vi "3DS Xray Beam.vi"(10 "FDD":sgl, 11 "DETECTOR SIZE":sgl) -> (3 "XRAY BEAM":T1 {"NormalList"."z" format="%.2f"; "NormalList"."y" format="%.2f"; "NormalList"."x" format="%.2f"; "VertexList"."z" format="%.2f"; "VertexList"."y" format="%.2f"; "VertexList"."x" format="%.2f"})   [LabVIEW 2026, in "XRay Beam.lvclass"]
uses:
  XRay Beam.lvclass
  <vilib>/picture/3D Picture Control/Old 3D Toolkit.llb/model.ctl
  <vilib>/picture/3D Picture Control/Old 3D Toolkit.llb/point3f.ctl
  <vilib>/picture/3D Picture Control/Old 3D Toolkit.llb/VertexMode.ctl
  <vilib>/picture/3D Picture Control/NI_Old 3D Toolkit.lvlib
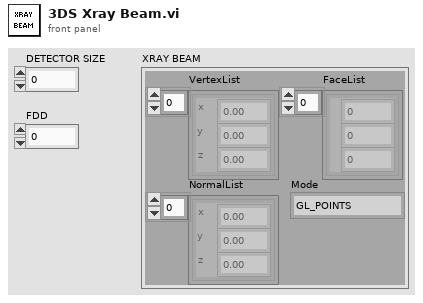
[diagram p1: front panel]
types:
  T1 = typedef "NI_3D Picture Control.lvlib/NI_Old 3D Toolkit.lvlib/model.ctl" = cluster{"VertexList":T2[], "FaceList":cluster{"v1":i32, "v2":i32, "v3":i32}[], "NormalList":T2[], "Mode":T3}
  T2 = typedef "NI_3D Picture Control.lvlib/NI_Old 3D Toolkit.lvlib/point3f.ctl" = cluster{"x":sgl, "y":sgl, "z":sgl}
  T3 = typedef "NI_3D Picture Control.lvlib/NI_Old 3D Toolkit.lvlib/VertexMode.ctl" = enum16{"GL_POINTS", "GL_LINES", "GL_LINE_LOOP", "GL_LINE_STRIP", "GL_TRIANGLES", "GL_TRIANGLE_STRIP", "GL_TRIANGLE_FAN", "GL_QUADS", "GL_QUAD_STRIP", "GL_POLYGON"}
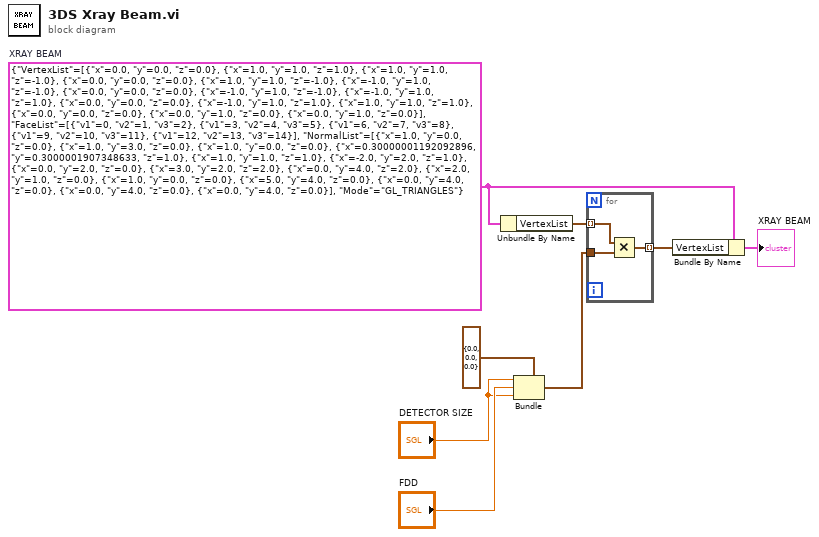
[diagram p0: block diagram]
diagram:
  w1 = T1 {"VertexList"=[{"x"=0.0, "y"=0.0, "z"=0.0}, {"x"=1.0, "y"=1.0, "z"=1.0}, {"x"=1.0, "y"=1.0, "z"=-1.0}, {"x"=0.0, "y"=0.0, "z"=0.0}, {"x"=1.0, "y"=1.0, "z"=-1.0}, {"x"=-1.0, "y"=1.0, "z"=-1.0}, {"x"=0.0, "y"=0.0, "z"=0.0}, {"x"=-1.0, "y"=1.0, "z"=-1.0}, {"x"=-1.0, "y"=1.0, "z"=1.0}, {"x"=0.0, "y"=0.0, "z"=0.0}, {"x"=-1.0, "y"=1.0, "z"=1.0}, {"x"=1.0, "y"=1.0, "z"=1.0}, {"x"=0.0, "y"=0.0, "z"=0.0}, {"x"=0.0, "y"=1.0, "z"=0.0}, {"x"=0.0, "y"=1.0, "z"=0.0}], "FaceList"=[{"v1"=0, "v2"=1, "v3"=2}, {"v1"=3, "v2"=4, "v3"=5}, {"v1"=6, "v2"=7, "v3"=8}, {"v1"=9, "v2"=10, "v3"=11}, {"v1"=12, "v2"=13, "v3"=14}], "NormalList"=[{"x"=1.0, "y"=0.0, "z"=0.0}, {"x"=1.0, "y"=3.0, "z"=0.0}, {"x"=1.0, "y"=0.0, "z"=0.0}, {"x"=0.3, "y"=0.3000002, "z"=1.0}, {"x"=1.0, "y"=1.0, "z"=1.0}, {"x"=-2.0, "y"=2.0, "z"=1.0}, {"x"=0.0, "y"=2.0, "z"=0.0}, {"x"=3.0, "y"=2.0, "z"=2.0}, {"x"=0.0, "y"=4.0, "z"=2.0}, {"x"=2.0, "y"=1.0, "z"=0.0}, {"x"=1.0, "y"=0.0, "z"=0.0}, {"x"=5.0, "y"=4.0, "z"=0.0}, {"x"=0.0, "y"=4.0, "z"=0.0}, {"x"=0.0, "y"=4.0, "z"=0.0}, {"x"=0.0, "y"=4.0, "z"=0.0}], "Mode"=enum."GL_TRIANGLES"}  # XRAY BEAM
  n1 = Unbundle By Name(w1) -> ("VertexList"=w4:T2[])
  n2 = Bundle(cluster=T2 {"x"=0.0, "y"=0.0, "z"=0.0} ("point3f"), "x"="DETECTOR SIZE", "y"="FDD", "z"="DETECTOR SIZE") -> (w5:T2)
  n3 = for {
    tunnel: w4 -> [w11] mode=indexing
    tunnel: w5 -> [w10]
    tunnel: [w9] -> w6 mode=indexing
    n4 = Multiply(x=w11, y=w10) -> (x*y=w9:T2)
  }
  n5 = Bundle By Name(cluster=w1, "VertexList"=w6) -> (→"XRAY BEAM":T1)
